vi "_RF.vi"(11 "RF":T1={"RF(GHz)"=880.0, "mm_multi(4or6)"=6.0, "SGPOUT(dBm)"=16.0, "SGGPIB"="29", "PAMP GPIB"="6", "VD (V)"=0.0, "VG (V)"=0.0, "multi (V)"=0.0} {"multi (V)" min=0.0 max=9.0 step=0.1; "VG (V)" min=0.0 max=4.0 step=0.1; "VD (V)" min=0.0 max=2.0 step=0.1}) -> ()   [LabVIEW 2017]
panel:
  out "SGfrq(GHz)":dbl=16.074074074074073
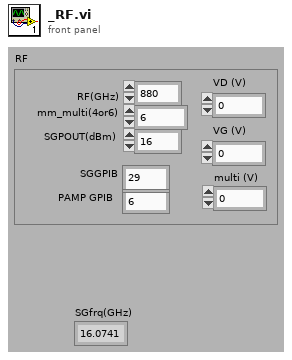
[diagram p1: front panel]
types:
  T1 = cluster{"RF(GHz)":dbl, "mm_multi(4or6)":dbl, "SGPOUT(dBm)":dbl, "SGGPIB":string, "PAMP GPIB":string, "VD (V)":dbl, "VG (V)":dbl, "multi (V)":dbl}
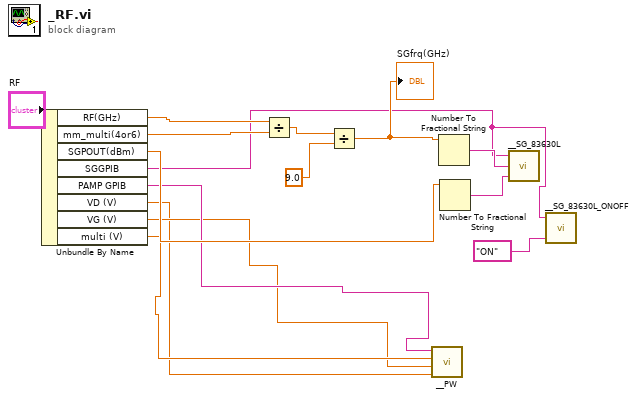
[diagram p0: block diagram]
diagram:
  n1 = Unbundle By Name("RF") -> ("RF(GHz)"=w9:dbl, "mm_multi(4or6)"=w8:dbl, "SGPOUT(dBm)"=w7:dbl, "SGGPIB"=w6:string, "PAMP GPIB"=w4:string, "VD (V)"=w1:dbl, "VG (V)"=w2:dbl, "multi (V)"=w3:dbl)
  n2 = Divide(x=w9, y=w8) -> (x/y=w15:dbl)
  n3 = Divide(x=w15, y=9.0) -> (x/y=w11:dbl)
  "SGfrq(GHz)" <- w11
  n4 = call "__PW.vi"("VC(V)"=w1, "VB(V)"=w2, "VA(V)"=w3, "GPIB"=w4) -> ()  [unwired: 5 in, 3 out]
  n5 = Number To Fractional String(number=w11) -> (F-format string=w13:string)  [unwired: 3 in]
  n6 = Number To Fractional String(number=w7) -> (F-format string=w12:string)  [unwired: 3 in]
  n7 = call "__SG_83630L.vi"("PW(dBm)"=w12, "frq(GHz)"=w13, "GPIB"=w6) -> ()
  n8 = call "__SG_83630L_ONOFF.vi"("ON/OFF"="ON", "GPIB"=w6) -> ()  [unwired: 1 in]
